vi "extrae puntos.vi"(11 "Array in":dbl[](array[numeric])) -> (1 "Curva de potencia":cluster{"Ramp Pattern":dbl[], dbl[]}(graph), 2 "Array out":dbl[](array[numeric]), 3 "Numero de puntos":i32)   [LabVIEW 2021]
uses:
  <vilib>/Analysis/1siggen.llb/Ramp Pattern by Delta.vi
  <vilib>/Analysis/NI_AALBase.lvlib
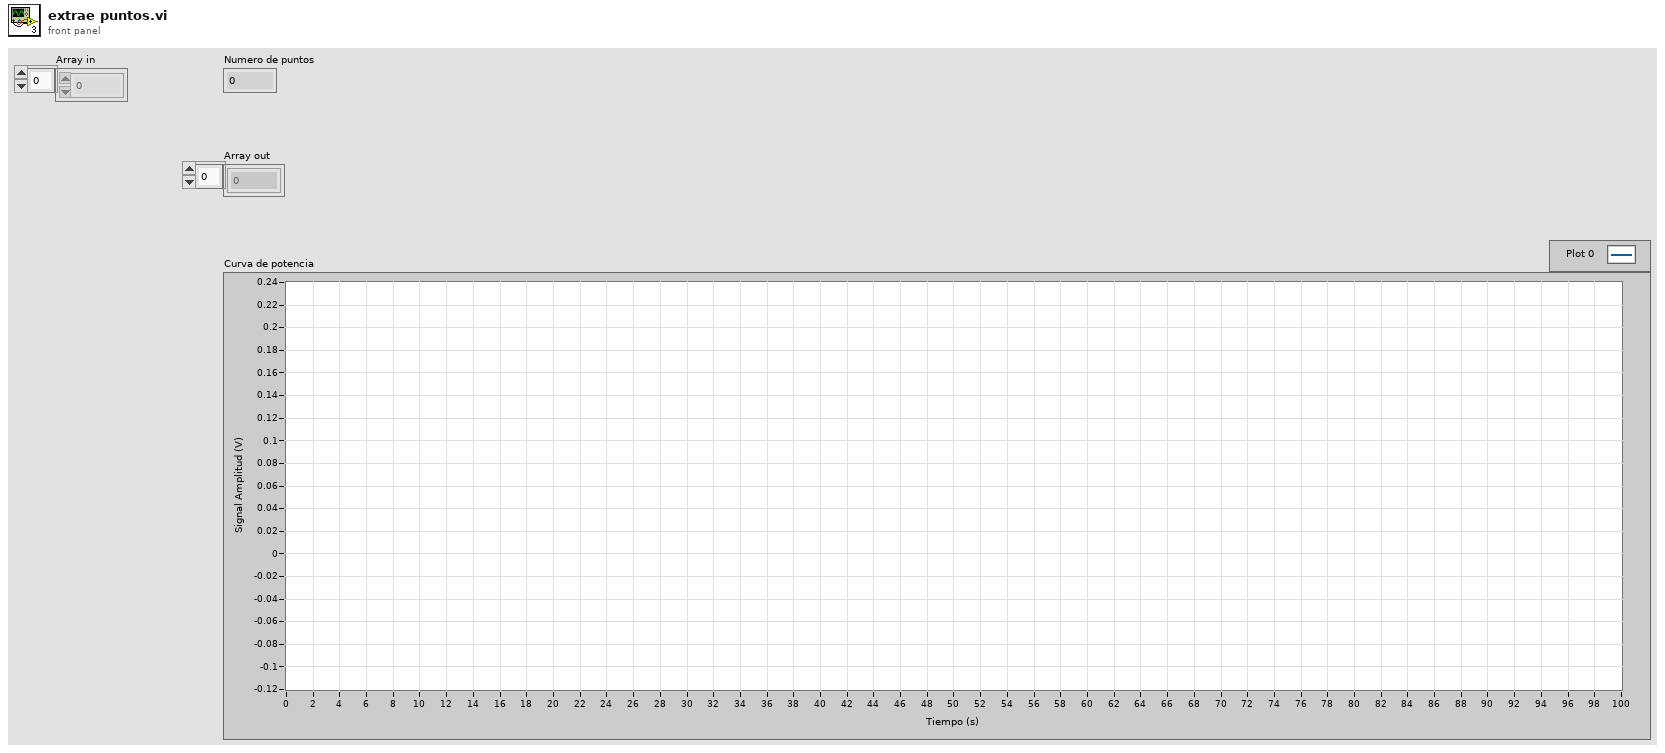
[diagram p1: front panel]
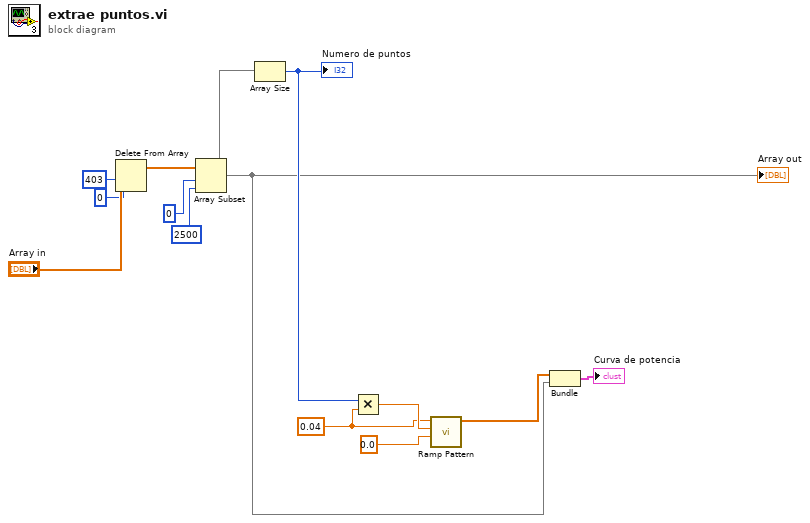
[diagram p0: block diagram]
diagram:
  w4 = 0.04 ("end")
  n1 = Delete From Array(array="Array in", length=403, index=0) -> (array with subset deleted=w10:dbl[])  [unwired: 1 out]
  n2 = Array Subset(array=w10, index=0, length=2500) -> (w2:dbl[])
  "Array out" <- w2
  n3 = Array Size(array=w2) -> (size(s)=w6:i32)
  "Numero de puntos" <- w6
  n4 = Multiply(x=w6, y=w4) -> (x*y=w5:dbl)
  n5 = call-poly <vilib>:"Ramp Pattern.vi"("start"=0.0 ("end"), "end"=w5, "delta"=w4) -> ("Ramp Pattern"=w3:dbl[])  [unwired: 6 in, 2 out]
  n6 = Bundle("Ramp Pattern"=w3, w2) -> (→"Curva de potencia":cluster{"Ramp Pattern":dbl[], dbl[]})  [unwired: 1 in]
